vi "Write Glue Reservoir.vi"(8 "error in (no error)":errorcluster, 10 "Glue Reservoir":T1, 11 "WorkTable Class in":refnum<class "WorkTable Class.lvclass">) -> (0 "error out":errorcluster, 3 "WorkTable Class out":refnum<class "WorkTable Class.lvclass">)   [LabVIEW 2011, in "WorkTable Class.lvclass"]
uses:
  WorkTable Class.lvclass
  Vec3d Class/Vec3d Class.lvclass
  WorkTable Class.lvclass/WorkTable Class.ctl
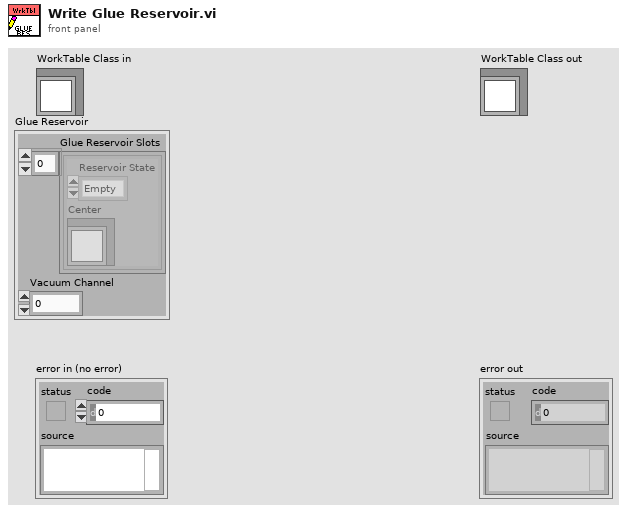
[diagram p1: front panel]
types:
  T1 = cluster{"Glue Reservoir Slots":cluster{"Reservoir State":enum16{"Empty", "Full", "Used"}, "Center":refnum<class "Vec3d Class.lvclass">}[], "Vacuum Channel":u8}
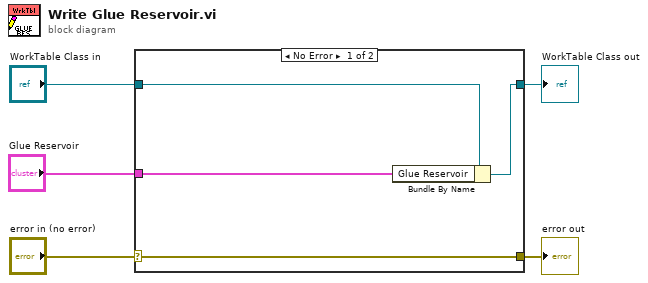
[diagram p0: block diagram]
diagram:
  n1 = case shown="No Error" "error in (no error)" {
    selector: "error in (no error)" -> [w9 w10]
    tunnel: [w9 w10] -> w4
    tunnel: [w7 w11] -> w2
    tunnel: "WorkTable Class in" -> [w8 w11]
    tunnel: "Glue Reservoir" -> [w6 _]
    frame No Error {
      n2 = Bundle By Name(cluster=w8, "Glue Reservoir"=w6) -> (w7:refnum<class "WorkTable Class.lvclass">)
    }
    frame Error {
    }
  }
  "error out" <- w4
  "WorkTable Class out" <- w2
